vi "dfd_FXP PtByPt Cascaded SOS Form II Transposed.vi"(0 "x":T1={"value"=0, "wl"=0, "iwl"=0, "Signed"=TRUE} {"value" format="%.0x"}, 1 "coef b":i64[](array[numeric]), 2 "coef a":i64[](array[numeric]), 3 "#sec":i32, 5 "filtering statistics in":T4(array[cluster]) {"statistics information"."min value" format="%.2f"; "statistics information"."max value" format="%.2f"; "Quantizer Source" items=["Coefficients a/k"=0, "Coefficients b/v"=7, "Input"=1, "Output"=2, "Multiplicand"=3, "Product"=4, "Sum"=5, "Delay"=6]}, 6 "FXPOPs":T5[](array[typedef]) {"source" items=["Coef a/k"=0, "Coef b/v"=7, "Input"=1, "Output"=2, "Multiplicand"=3, "Product"=4, "Sum"=5, "Delay"=6, "Gain"=8]}, 7 "state in":i64[](array[numeric])) -> (13 "state out":i64[](array[numeric]), 14 "filtered x":T1={"value"=0, "wl"=0, "iwl"=0, "Signed"=TRUE} {"value" format="%.0x"}, 19 "filtering statistics out":T4(array[cluster]) {"statistics information"."min value" format="%.2f"; "statistics information"."max value" format="%.2f"; "Quantizer Source" items=["Coefficients a/k"=0, "Coefficients b/v"=7, "Input"=1, "Output"=2, "Multiplicand"=3, "Product"=4, "Sum"=5, "Delay"=6]})   [LabVIEW 2017, in "NI_DigFilter_FXP.lvlib"]
uses:
  <vilib>/addons/Digital Filter Design/NI_DigFilter_FXP.lvlib
  <vilib>/addons/Digital Filter Design/_Objects.llb/dfd_DFXP Data Type (scaler).ctl
  <vilib>/addons/Digital Filter Design/_Objects.llb/dfd_DFXP Operation Parameter.ctl
  <vilib>/addons/Digital Filter Design/_Objects.llb/dfd_Internal Quantization Srcs.ctl
  <vilib>/addons/Digital Filter Design/_Objects.llb/DFD Quantization Sources.ctl
  <vilib>/addons/Digital Filter Design/_Objects.llb/DFD FXP Statistics Data.ctl
  <vilib>/addons/Digital Filter Design/NI_DigFilterLicensed.lvlib
panel:
  in  "coef_a":T1={"value"=0, "wl"=0, "iwl"=0, "Signed"=TRUE} {"value" format="%.0x"}
  in  "coef_b":T1={"value"=0, "wl"=0, "iwl"=0, "Signed"=TRUE} {"value" format="%.0x"}
  in  "state":T1={"value"=0, "wl"=0, "iwl"=0, "Signed"=TRUE} {"value" format="%.0x"}
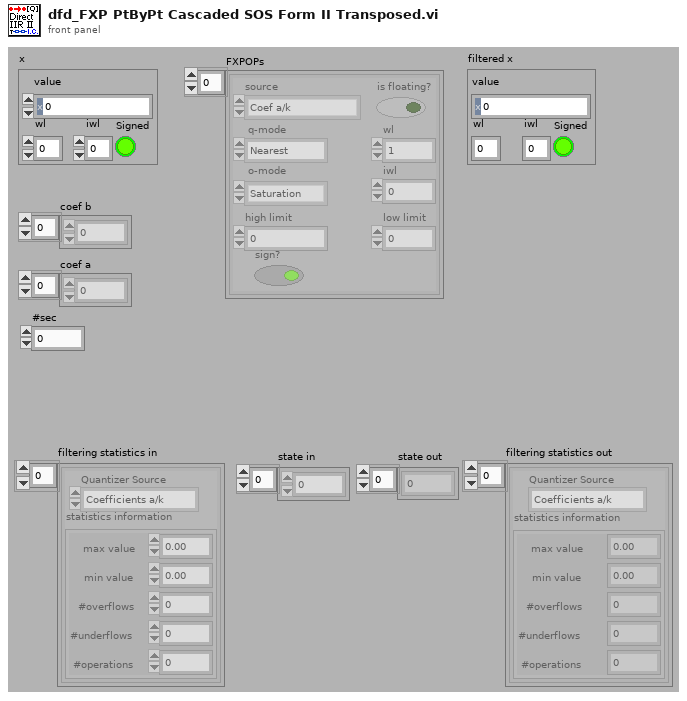
[diagram p1: front panel]
types:
  T1 = typedef "dfd_DFXP Data Type (scaler).ctl" = cluster{"value":i64, "wl":i16, "iwl":i16, "Signed":bool}
  T2 = typedef "NI_DigFilterLicensed.lvlib/DFD Quantization Sources.ctl" = u16
  T3 = typedef "NI_DigFilterLicensed.lvlib/DFD FXP Statistics Data.ctl" = cluster{"max value":ext, "min value":ext, "#overflows":i32, "#underflows":i32, "#operations":i32}
  T4 = cluster{"Quantizer Source":T2, "statistics information":T3}[]
  T5 = typedef "dfd_DFXP Operation Parameter.ctl" = cluster{"source":T6, "is floating?":bool, "o-mode":enum16{"Saturation", "Wrap"}, "q-mode":enum16{"Nearest", "Truncation"}, "wl":i16, "high limit":i64, "low limit":i64, "iwl":i16, "sign?":bool}
  T6 = typedef "NI_DigFilterLicensed.lvlib/dfd_Internal Quantization Srcs.ctl" = u16
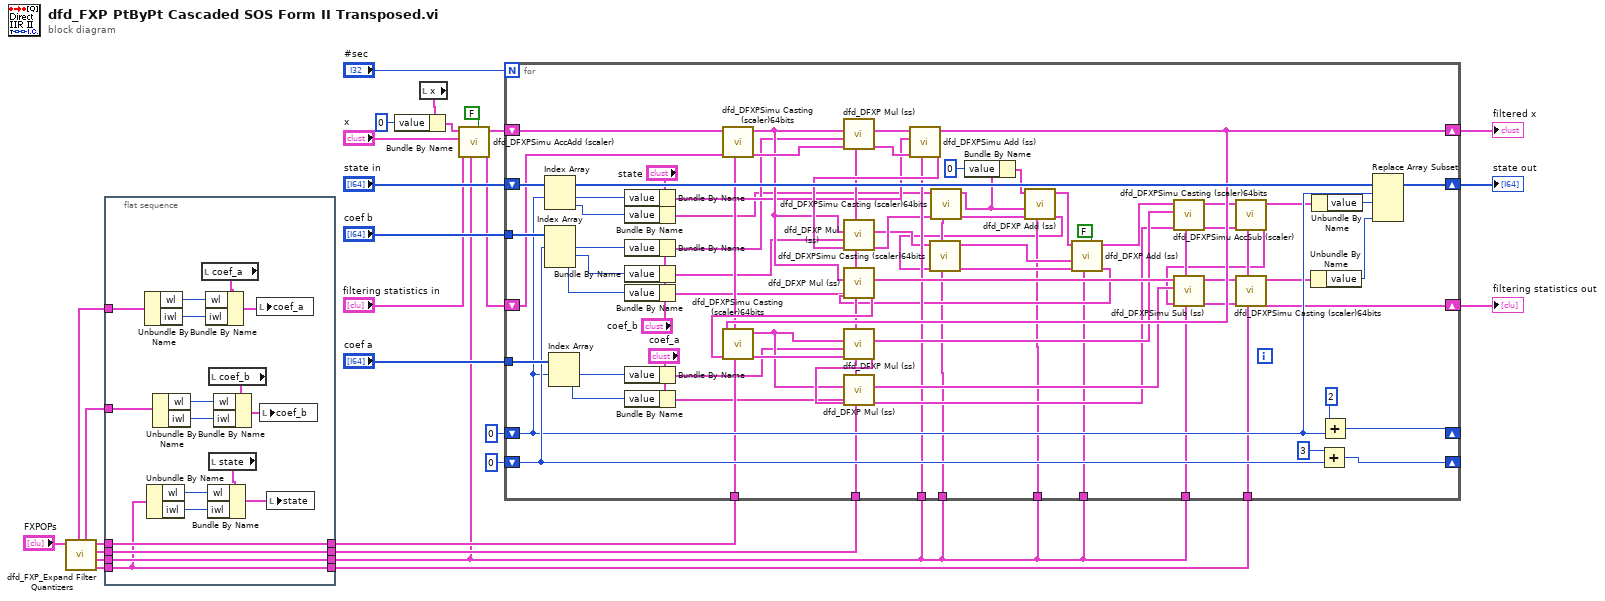
[diagram p0: block diagram]
diagram:
  n1 = call <vilib>:"dfd_FXP_Expand Filter Quantizers.vi"("FXPOPs"="FXPOPs") -> ("Delay"=w10:T5, "Sum"=w11:T5, "Product"=w12:T5, "Multiplicand"=w13:T5, "Coefficient b/v"=w5:T5, "Coefficient a/k"=w6:T5)  [unwired: 5 out]
  n2 = flat-sequence {
    tunnel: w10 -> [w29]
    tunnel: w13 -> [w42]
    tunnel: [w42] -> w9
    tunnel: [w41] -> w8
    tunnel: w12 -> [w41]
    tunnel: w11 -> [w40]
    tunnel: [w40] -> w1
    tunnel: [w29] -> _
    tunnel: w5 -> [w38]
    tunnel: w6 -> [w32]
    tunnel: [w29] -> w7
    frame #0 {
      n3 = Unbundle By Name(w32) -> ("wl"=w34:i16, "iwl"=w33:i16)
      n4 = Unbundle By Name(w29) -> ("wl"=w45:i16, "iwl"=w44:i16)
      n5 = Unbundle By Name(w38) -> ("wl"=w35:i16, "iwl"=w39:i16)
      n6 = local read "coef_a"() -> (w30:T1)
      n7 = Bundle By Name(cluster=w30, "wl"=w34, "iwl"=w33) -> (w31:T1)
      n8 = local read "coef_b"() -> (w36:T1)
      n9 = local read "state"() -> (w46:T1)
      n10 = Bundle By Name(cluster=w46, "wl"=w45, "iwl"=w44) -> (w43:T1)
      n11 = Bundle By Name(cluster=w36, "wl"=w35, "iwl"=w39) -> (w37:T1)
      n12 = local write "coef_a"(w31) -> ()
      n13 = local write "coef_b"(w37) -> ()
      n14 = local write "state"(w43) -> ()
    }
  }
  n15 = local read "x"() -> (w4:T1)
  n16 = Bundle By Name(cluster=w4, "value"=i64 0) -> (w2:T1)
  n17 = call <vilib>:"dfd_DFXPSimu AccAdd (scaler).vi"("quantize output? (T)"=FALSE ("quantize output?"), "op params"=w1, "filtering statistics in"="filtering statistics in", "addend"="x", "acc in"=w2) -> ("filtering statistics out"=w15:T4, "acc out"=w17:T1)  [unwired: 5 out]
  n18 = for {
    N: "#sec" -> [_]
    shift-right: [w119] -> w27
    shift-left: "state in" -> [w120]
    shift-right: [w118] -> _
    shift-left: 0 -> [w111]
    shift-right: [w104] -> w21
    shift-left: w17 -> [w108]
    shift-right: [w115] -> _
    shift-left: 0 -> [w112]
    tunnel: "coef b" -> [w114]
    tunnel: "coef a" -> [w113]
    tunnel: w9 -> [w92]
    tunnel: w8 -> [w91]
    tunnel: w1 -> [w73]
    tunnel: w1 -> [w90]
    tunnel: w7 -> [w89]
    shift-right: [w93] -> w19
    shift-left: w15 -> [w101]
    tunnel: w1 -> [w88]
    tunnel: w1 -> [w56]
    tunnel: w1 -> [w48]
    n19 = Index Array(array=w120, index #1=w111) -> (element #1=w106:i64, element #2=w71:i64)  [unwired: 1 in]
    n20 = Index Array(array=w114, index #1=w112) -> (element #1=w87:i64, element #2=w86:i64, element #3=w84:i64)  [unwired: 2 in]
    n21 = Index Array(array=w113, index #1=w111) -> (element #1=w83:i64, element #2=w81:i64)  [unwired: 1 in]
    n22 = Bundle By Name(cluster="state", "value"=w106) -> (w70:T1)
    n23 = Bundle By Name(cluster="state", "value"=w71) -> (w59:T1)
    n24 = Bundle By Name(cluster="coef_b", "value"=w87) -> (w69:T1)
    n25 = Bundle By Name(cluster="coef_b", "value"=w86) -> (w68:T1)
    n26 = Bundle By Name(cluster="coef_b", "value"=w84) -> (w67:T1)
    n27 = Bundle By Name(cluster="coef_a", "value"=w83) -> (w65:T1)
    n28 = Bundle By Name(cluster="coef_a", "value"=w81) -> (w64:T1)
    n29 = call <vilib>:"dfd_DFXPSimu Casting (scaler)64bits.vi"("op params"=w92, "filtering statistics in"=w101, "Value in"=w108) -> ("filtering statistics out"=w100:T4, "Value out"=w85:T1)  [unwired: 2 in, 5 out]
    n30 = call <vilib>:"dfd_DFXP Mul (ss).vi"("op params"=w91, "filtering statistics in"=w100, "Value in 2"=w69, "Value in"=w85) -> ("filtering statistics out"=w99:T4, "Value out"=w107:T1)  [unwired: 6 out]
    n31 = call <vilib>:"dfd_DFXPSimu Add (ss).vi"("op params"=w88, "filtering statistics in"=w99, "value in 2"=w70, "value in 1"=w107) -> ("filtering statistics out"=w98:T4, "value out"=w104:T1)  [unwired: 1 in, 5 out]
    n32 = call <vilib>:"dfd_DFXP Mul (ss).vi"("op params"=w91, "filtering statistics in"=w98, "Value in 2"=w68, "Value in"=w85) -> ("filtering statistics out"=w58:T4, "Value out"=w57:T1)  [unwired: 6 out]
    n33 = call <vilib>:"dfd_DFXPSimu Casting (scaler)64bits.vi"("op params"=w56, "filtering statistics in"=w58, "Value in"=w59) -> ("filtering statistics out"=w52:T4, "Value out"=w50:T1)  [unwired: 1 in, 6 out]
    n34 = Bundle By Name(cluster=w50, "value"=i64 0) -> (w49:T1)
    n35 = call <vilib>:"dfd_DFXP Add (ss).vi"("op params"=w48, "filtering statistics in"=w52, "Value in 2"=w50, "Value in"=w49) -> ("filtering statistics out"=w47:T4, "Value out"=w53:T1)  [unwired: 1 in, 5 out]
    n36 = call <vilib>:"dfd_DFXPSimu Casting (scaler)64bits.vi"("op params"=w56, "filtering statistics in"=w47, "Value in"=w57) -> ("filtering statistics out"=w54:T4, "Value out"=w55:T1)  [unwired: 1 in, 6 out]
    n37 = call <vilib>:"dfd_DFXP Add (ss).vi"("quantize output? (T)"=FALSE ("quantize output?"), "op params"=w73, "filtering statistics in"=w54, "Value in 2"=w55, "Value in"=w53) -> ("filtering statistics out"=w74:T4, "Value out"=w75:T1)  [unwired: 5 out]
    n38 = call <vilib>:"dfd_DFXP Mul (ss).vi"("op params"=w91, "filtering statistics in"=w74, "Value in 2"=w67, "Value in"=w85) -> ("filtering statistics out"=w97:T4, "Value out"=w105:T1)  [unwired: 6 out]
    n39 = call <vilib>:"dfd_DFXPSimu Casting (scaler)64bits.vi"("op params"=w92, "filtering statistics in"=w97, "Value in"=w104) -> ("filtering statistics out"=w96:T4, "Value out"=w82:T1)  [unwired: 2 in, 5 out]
    n40 = call <vilib>:"dfd_DFXP Mul (ss).vi"("op params"=w91, "filtering statistics in"=w96, "Value in 2"=w65, "Value in"=w82) -> ("filtering statistics out"=w95:T4, "Value out"=w103:T1)  [unwired: 6 out]
    n41 = call <vilib>:"dfd_DFXP Mul (ss).vi"("op params"=w91, "filtering statistics in"=w95, "Value in 2"=w64, "Value in"=w82) -> ("filtering statistics out"=w94:T4, "Value out"=w102:T1)  [unwired: 6 out]
    n42 = call <vilib>:"dfd_DFXPSimu AccSub (scaler).vi"("op params"=w90, "filtering statistics in"=w94, "addend"=w103, "acc in"=w75) -> ("filtering statistics out"=w78:T4, "acc out"=w79:T1)  [unwired: 2 in, 4 out]
    n43 = call <vilib>:"dfd_DFXPSimu Casting (scaler)64bits.vi"("op params"=w89, "filtering statistics in"=w78, "Value in"=w79) -> ("filtering statistics out"=w77:T4, "Value out"=w109:T1)  [unwired: 2 in, 5 out]
    n44 = call <vilib>:"dfd_DFXPSimu Sub (ss).vi"("op params"=w90, "filtering statistics in"=w77, "value in 2"=w102, "value in 1"=w105) -> ("filtering statistics out"=w76:T4, "value out"=w80:T1)  [unwired: 1 in, 5 out]
    n45 = call <vilib>:"dfd_DFXPSimu Casting (scaler)64bits.vi"("op params"=w89, "filtering statistics in"=w76, "Value in"=w80) -> ("filtering statistics out"=w93:T4, "Value out"=w110:T1)  [unwired: 2 in, 5 out]
    n46 = Unbundle By Name(w110) -> ("value"=w62:i64)
    n47 = Unbundle By Name(w109) -> ("value"=w61:i64)
    n48 = Add(x=3, y=w112) -> (x+y=w115:i32)
    n49 = Add(x=2 ("y"), y=w111) -> (x+y=w118:i32)
    n50 = Replace Array Subset(array=w120, new element #1=w61, index #1=w111, new element #2=w62) -> (w119:i64[])  [unwired: 1 in]
  }
  "filtered x" <- w21
  "state out" <- w27
  "filtering statistics out" <- w19
